vi "AuMT8852B AFH Pseudo Local Assessment Map.vi"(5 "Hex Representation of Map":string, 7 "Pseudo Map":cluster{"Pseudo Local Assessment Map":bool[][]} caption="Pseudo Local Assessment Map", 8 "error in (no error)":errorcluster, 10 "Generate Map (Use Map)":enum16{"Use map", "Use hex string"}(ring), 11 "VISA session":refnum<visa-resource-name>) -> (0 "error out":errorcluster, 2 "error code":i32, 3 "VISA session out":refnum<visa-resource-name>)   [LabVIEW 2017]
doc: "Anritsu MT8852B Bluetooth Tester\n\nConfigures the Pseudo Local Assessment Map.\n\nINPUTS\nPseudo Local Assessment Map - configures the map on the instrument according to the channels enabled on this control.\nHex Representation of map - the hexadecimal representation of the pseudo local assessment map converted from the channel map or entered by the user."
panel:
  # "0"
  # "10"
  # "20"
  # "30"
  # "40"
  # "50"
  # "60"
  # "70"
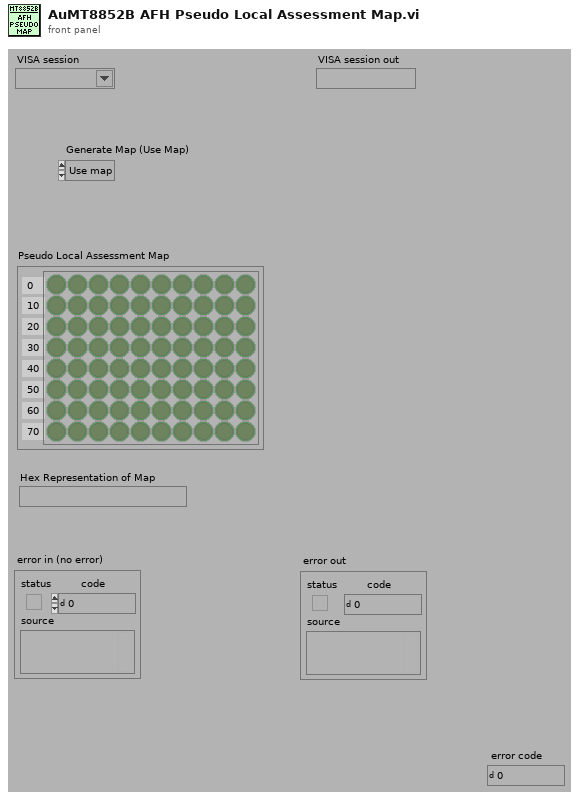
[diagram p1: front panel]
types:
  T1 = enum16{"Simulate", "Range check", "Cache", "Query instrument status"}
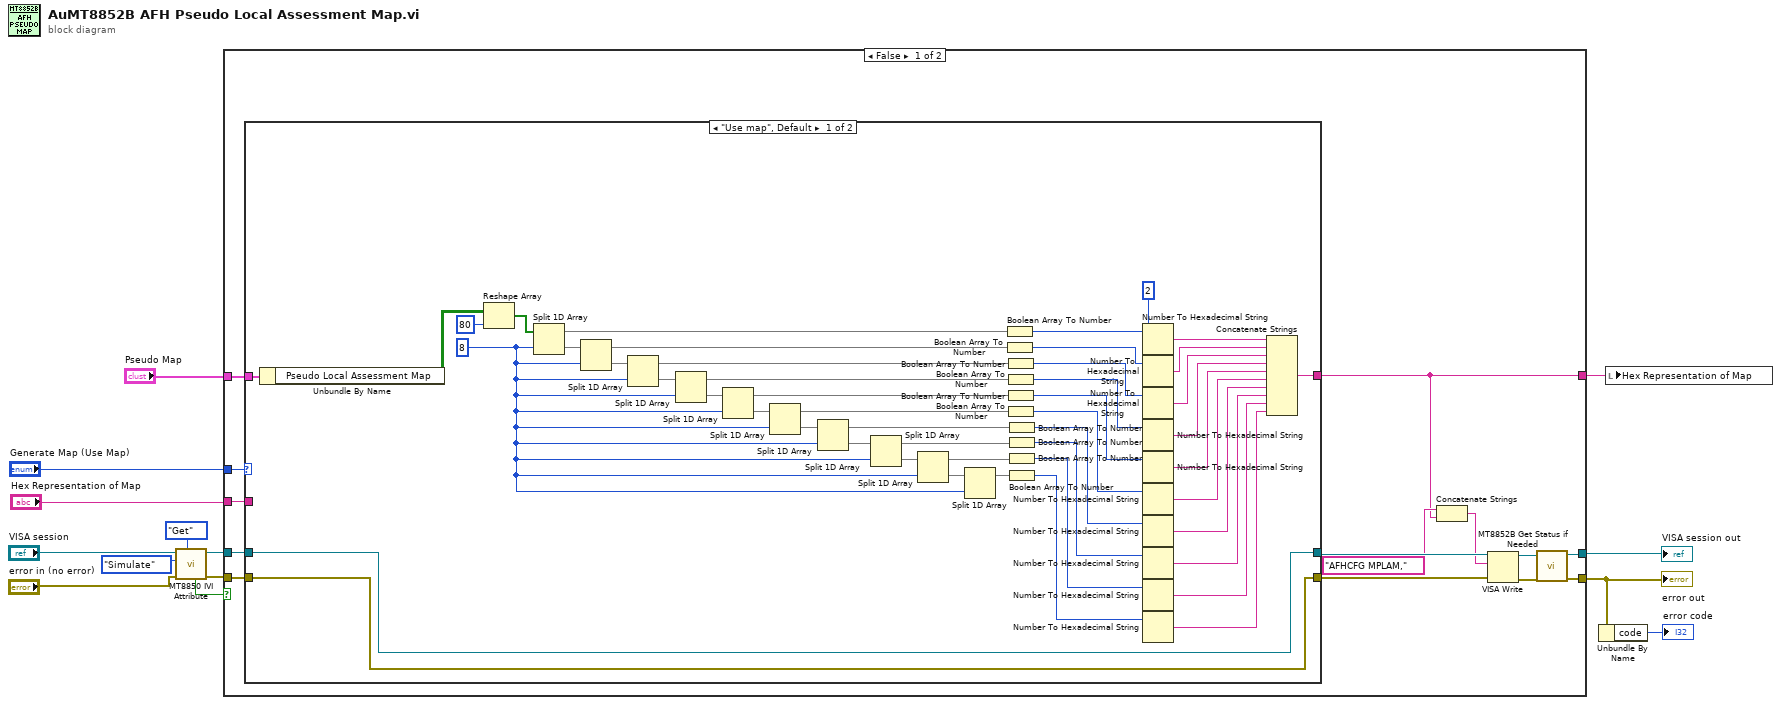
[diagram p0: block diagram]
diagram:
  n1 = call <instrlib>:"MT8850 IVI Attribute.vi"("Set/Get (Set)"=enum16{"Set", "Get"}."Get", "error in (no error)"="error in (no error)", "Flag (Simulate)"=T1."Simulate", "VISA session"="VISA session") -> ("error out"=w13:errorcluster, "VISA session out"=w14:refnum<visa-resource-name>, "Value out"=w10:bool)  [unwired: 5 in]
  n2 = case shown="False" w10 {
    tunnel: [w20 w82] -> w8
    tunnel: [w28 w81] -> w7
    tunnel: w14 -> [w23 w82]
    tunnel: w13 -> [w26 w81]
    tunnel: "Generate Map (Use Map)" -> [w27 _]
    tunnel: "Hex Representation of Map" -> [w17 w80]
    tunnel: [w16 w80] -> w2
    tunnel: "Pseudo Map" -> [w15 _]
    frame False {
      n3 = case shown="\"Use map\", Default" w27 {
        tunnel: [w34 w77] -> w16
        tunnel: w26 -> [w33 w79]
        tunnel: [w33 w79] -> w25
        tunnel: [w32 w78] -> w24
        tunnel: w23 -> [w32 w78]
        tunnel: w17 -> [_ w77]
        tunnel: w15 -> [w31 _]
        frame "Use map", Default {
          w29 = i16 2 ("width (-)")
          w65 = 8
          n4 = Unbundle By Name(w31) -> ("Pseudo Local Assessment Map"=w30:bool[][])
          n5 = Reshape Array(w30, 80 ("dimension size")) -> (w75:bool[])
          n6 = Split 1D Array(array=w75, index=w65) -> (first subarray=w64:bool[], second subarray=w74:bool[])
          n7 = Split 1D Array(array=w74, index=w65) -> (first subarray=w63:bool[], second subarray=w73:bool[])
          n8 = Split 1D Array(array=w73, index=w65) -> (first subarray=w62:bool[], second subarray=w70:bool[])
          n9 = Split 1D Array(array=w70, index=w65) -> (first subarray=w61:bool[], second subarray=w72:bool[])
          n10 = Split 1D Array(array=w72, index=w65) -> (first subarray=w60:bool[], second subarray=w71:bool[])
          n11 = Split 1D Array(array=w71, index=w65) -> (first subarray=w59:bool[], second subarray=w69:bool[])
          n12 = Split 1D Array(array=w69, index=w65) -> (first subarray=w58:bool[], second subarray=w68:bool[])
          n13 = Split 1D Array(array=w68, index=w65) -> (first subarray=w57:bool[], second subarray=w67:bool[])
          n14 = Split 1D Array(array=w67, index=w65) -> (first subarray=w56:bool[], second subarray=w66:bool[])
          n15 = Split 1D Array(array=w66, index=w65) -> (first subarray=w55:bool[])  [unwired: 1 out]
          n16 = Boolean Array To Number(Boolean array=w64) -> (number=w54:u32)
          n17 = Boolean Array To Number(Boolean array=w63) -> (number=w53:u32)
          n18 = Boolean Array To Number(Boolean array=w62) -> (number=w52:u32)
          n19 = Boolean Array To Number(Boolean array=w61) -> (number=w51:u32)
          n20 = Boolean Array To Number(Boolean array=w60) -> (number=w50:u32)
          n21 = Boolean Array To Number(Boolean array=w59) -> (number=w49:u32)
          n22 = Boolean Array To Number(Boolean array=w58) -> (number=w48:u32)
          n23 = Boolean Array To Number(Boolean array=w57) -> (number=w47:u32)
          n24 = Boolean Array To Number(Boolean array=w56) -> (number=w46:u32)
          n25 = Boolean Array To Number(Boolean array=w55) -> (number=w45:u32)
          n26 = Number To Hexadecimal String(1:w29, 2:w54) -> (0:w44:string)
          n27 = Number To Hexadecimal String(1:w29, 2:w53) -> (0:w43:string)
          n28 = Number To Hexadecimal String(1:w29, 2:w52) -> (0:w42:string)
          n29 = Number To Hexadecimal String(1:w29, 2:w51) -> (0:w41:string)
          n30 = Number To Hexadecimal String(1:w29, 2:w50) -> (0:w40:string)
          n31 = Number To Hexadecimal String(1:w29, 2:w49) -> (0:w39:string)
          n32 = Number To Hexadecimal String(1:w29, 2:w48) -> (0:w38:string)
          n33 = Number To Hexadecimal String(1:w29, 2:w47) -> (0:w37:string)
          n34 = Number To Hexadecimal String(1:w29, 2:w46) -> (0:w36:string)
          n35 = Number To Hexadecimal String(1:w29, 2:w45) -> (0:w35:string)
          n36 = Concatenate Strings(w44, w43, w42, w41, w40, w39, w38, w37, w36, w35) -> (w34:string)
        }
        frame "Use hex string" {
        }
      }
      n37 = Concatenate Strings("AFHCFG MPLAM,", w16) -> (w19:string)
      n38 = VISA Write(VISA resource name=w24, write buffer=w19, error in (no error)=w25) -> (VISA resource name out=w21:refnum<visa-resource-name>, error out=w22:errorcluster)  [unwired: 1 out]
      n39 = call <instrlib>:"MT8852B Get Status if Needed.vi"("error in (no error)"=w22, "VISA session"=w21) -> ("error out"=w28:errorcluster, "VISA session out"=w20:refnum<visa-resource-name>)  [unwired: 8 in]
    }
    frame True {
    }
  }
  "error out" <- w7
  "VISA session out" <- w8
  n40 = Unbundle By Name(w7) -> ("code"=→"error code":i32)
  n41 = local write "Hex Representation of Map"(w2) -> ()
